vi "Data File Header Constants.vi"() -> ()   [LabVIEW 2023, in "File IO.lvclass"]
uses:
  File IO.lvclass
panel:
  out "Data end divider":string="****"
  out "Header end divider":string="===================="
  out "Header start divider":string="--------------------"
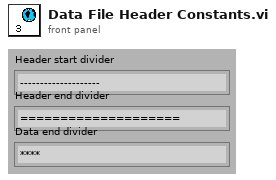
[diagram p1: front panel]
diagram:
